vi "Test Position INI.vi"(11 "Test Case In":refnum<class "Editor Position.lvclass">) -> (0 "error out":errorcluster, 3 "Test Case Out":refnum<class "Editor Position.lvclass">)   [LabVIEW 2021, in "Editor Position.lvclass"]
doc: "Tests the reading from and writing to the INI file."
uses:
  Editor Position.lvclass
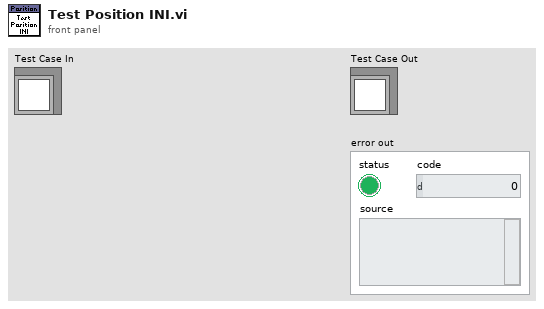
[diagram p1: front panel]
types:
  T1 = cluster{"Position Value":string, "Position Existed":bool, "Use Size Value":bool, "Use Size Existed":bool}
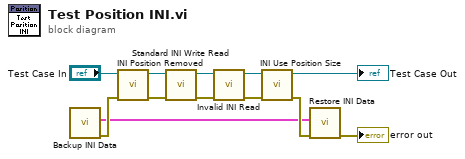
[diagram p0: block diagram]
diagram:
  n1 = call "Backup INI Data.vi"() -> ("error out"=w11:errorcluster, "INI Data Backup"=w6:T1)  [unwired: 10 in]
  n2 = call "INI Position Removed.vi"("error in"=w11, "Editor Position in"="Test Case In") -> ("error out"=w10:errorcluster, "Editor Position out"=w4:refnum<class "Editor Position.lvclass">)  [unwired: 8 in]
  n3 = call "Standard INI Write Read.vi"("error in"=w10, "Editor Position in"=w4) -> ("error out"=w9:errorcluster, "Editor Position out"=w3:refnum<class "Editor Position.lvclass">)  [unwired: 8 in]
  n4 = call "Invalid INI Read.vi"("error in"=w9, "Editor Position in"=w3) -> ("error out"=w8:errorcluster, "Editor Position out"=w2:refnum<class "Editor Position.lvclass">)  [unwired: 8 in]
  n5 = call "INI Use Position Size.vi"("error in"=w8, "Editor Position in"=w2) -> ("error out"=w7:errorcluster, "Editor Position out"=→"Test Case Out":refnum<class "Editor Position.lvclass">)  [unwired: 8 in]
  n6 = call "Restore INI Data.vi"("error in"=w7, "INI Data Backup"=w6) -> ("error out"=→"error out":errorcluster)  [unwired: 9 in]
